vi "Configure_Voltage.vi"(8 "error in (no error)":errorcluster, 10 "DC_Voltage_Configuration":variant, 11 "Measure_Voltage in":refnum<class "Measure_Voltage.lvclass">) -> (0 "error out":errorcluster, 3 "Measure_Voltage out":refnum<class "Measure_Voltage.lvclass">)   [LabVIEW 2020, in "Measure_Voltage.lvclass"]
uses:
  Measure_Voltage.lvclass
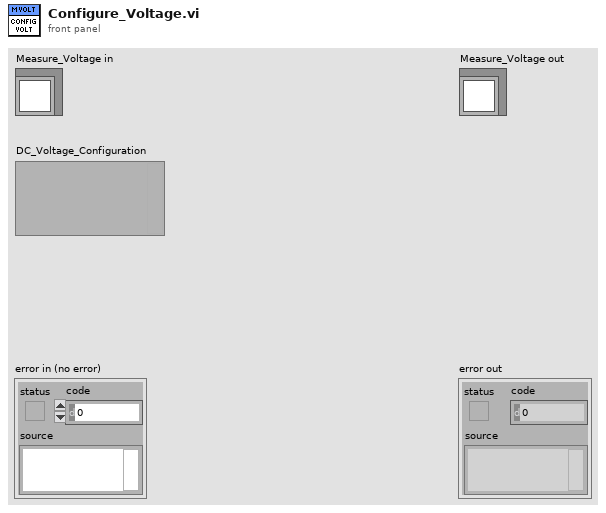
[diagram p1: front panel]
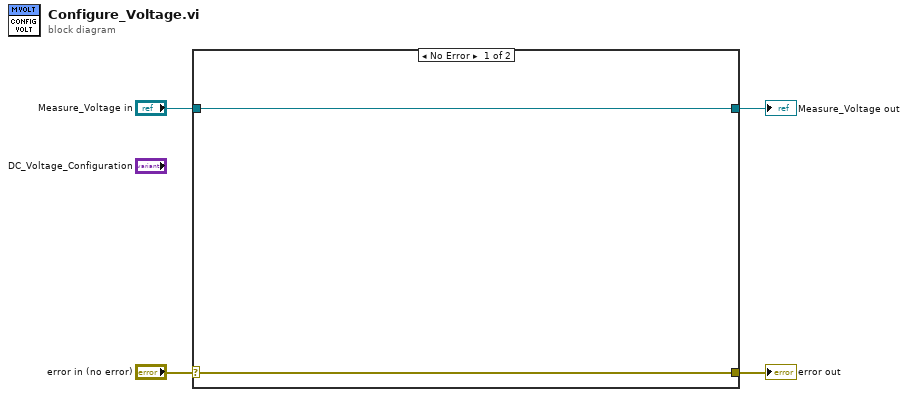
[diagram p0: block diagram]
diagram:
  n1 = case shown="No Error" "error in (no error)" {
    selector: "error in (no error)" -> [w5 w8]
    tunnel: [w5 w8] -> w3
    tunnel: [w6 w7] -> w1
    tunnel: "Measure_Voltage in" -> [w6 w7]
    frame No Error {
    }
    frame Error {
    }
  }
  "error out" <- w3
  "Measure_Voltage out" <- w1
